vi "Fetch.vi"(8 "error in (no error)":errorcluster, 10 "Message in":refnum<class "FetchMessage.lvclass">, 11 "RSA in":refnum<class "RSA.lvclass">) -> (0 "error out":errorcluster, 3 "RSA out":refnum<class "RSA.lvclass">)   [LabVIEW 2012, in "RSA.lvclass"]
doc: "The fetch method processes the command 'fetch'.\n\nThe command 'fetch' is used for receiving various forms of data."
uses:
  RSA.lvclass
  <vilib>/Distrio/Murmex/FetchMessage/FetchMessage.lvclass
  <vilib>/Distrio/Murmex/Murmex/Murmex.lvclass
panel:
  # "This method is called when the FETCH\ntrigger is sent. \n\nOverride this method when your component needs to\nrespond to this trigger. \n\nCall parent for proper implementation"
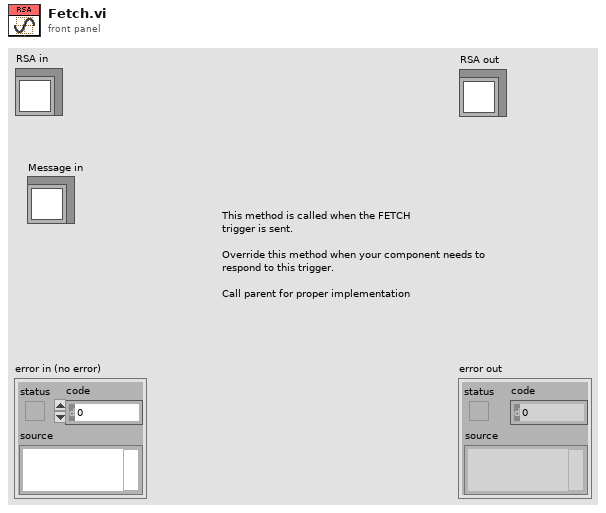
[diagram p1: front panel]
types:
  T1 = typedef "Murmex.lvlib/FetchMessage.lvclass/Channel data cluster.ctl" = cluster{"channel id":i32, "data UInt8":u8[], "data type":T2, "dimensions":i32[], "physical units":T3[], "waveform dt":dbl, "waveform":T4}
  T2 = typedef "Murmex.lvlib/Murmex.lvclass/data_type_enum.ctl" = enum16{"Float128", "Float64", "Float32", "Int64", "Int32", "Int16", "Int8", "UInt64", "UInt32", "UInt16", "UInt8", "Boolean", "String"}
  T3 = typedef "Physical Units__ogtk.ctl" = cluster{"Base Units":enum16{"radian", "steradian", "second", "meter", "kilogram", "ampere", "kelvin", "mole", "candela"}, "Exponent":i16}
  T4 = typedef "Murmex.lvlib/Murmex.lvclass/waveform_type_enum.ctl" = enum16{"no waveform", "analog", "digital"}
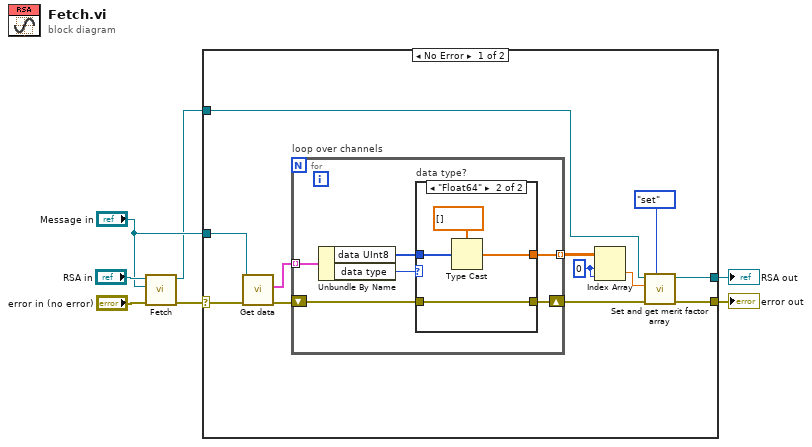
[diagram p0: block diagram]
diagram:
  n1 = call-parent "Fetch.vi"("error in (no error)"="error in (no error)", "Message in"="Message in", "Murmex in"="RSA in") -> ("error out"=w5:errorcluster, "Murmex out"=w3:refnum<class "RSA.lvclass">)  [unwired: 7 in]
  n2 = case shown="No Error" w5 {
    selector: w5 -> [w17 w32]
    tunnel: "Message in" -> [w16 _]
    tunnel: w3 -> [w9 w31]
    tunnel: [w10 w32] -> w2
    tunnel: [w8 w31] -> w1
    frame No Error {
      w14 = 0 ("index (row)")
      n3 = call <vilib>:"Get data.vi"("error in (no error)"=w17, "FetchMessage.lvclass"=w16) -> ("error out"=w18:errorcluster, "data (channels)"=w19:T1[])  [unwired: 7 in, 1 out]
      n4 = for "loop over channels" {
        tunnel: w19 -> [w23] mode=indexing
        shift-right: [w21] -> w12
        shift-left: w18 -> [w22]
        tunnel: [w20] -> w15 mode=indexing
        n5 = Unbundle By Name(w23) -> ("data UInt8"=w25:u8[], "data type"=w24:T2)
        n6 = case "data type?" shown="\"Float64\"" w24 {
          tunnel: w25 -> [_ w30]
          tunnel: [_ w29] -> w20
          tunnel: w22 -> [w26 w27]
          tunnel: [w26 w27] -> w21
          frame Default {
          }
          frame "Float64" {
            n7 = Type Cast(type=dbl[] [] ("run time Cluster.1x160 Voltage Map"), x=w30) -> (*(type *) &x=w29:dbl[])
          }
        }
      }
      n8 = Index Array(array=w15, index (row)=w14, index (col)=w14) -> (element=w11:dbl)
      n9 = call "Set and get merit factor array.vi"("action"=enum16{"set", "get", "initialise"}."set", "error in (no error)"=w12, "merit factor"=w11, "RSA in"=w9) -> ("error out"=w10:errorcluster, "RSA out"=w8:refnum<class "RSA.lvclass">)  [unwired: 4 in, 2 out]
    }
    frame Error {
    }
  }
  "error out" <- w2
  "RSA out" <- w1
